vi "Unsubscribe.vi"(8 "error in (no error)":errorcluster, 11 "Subscription":refnum<class "Subscription.lvclass">) -> (0 "error out":errorcluster)   [LabVIEW 2015, in "NI_AWS_SNS.lvlib" / "Subscription.lvclass"]
doc: "Deletes a subscription.\n\nThis action is throttled at 100 transactions per second (TPS)."
uses:
  Subscription.lvclass
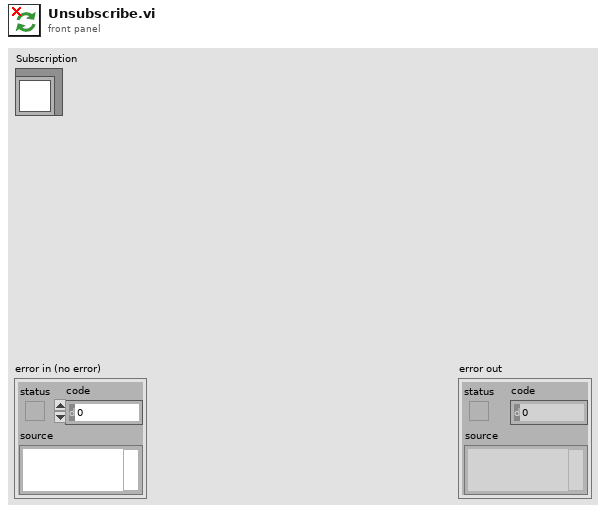
[diagram p1: front panel]
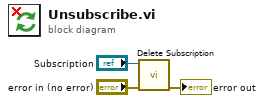
[diagram p0: block diagram]
diagram:
  n1 = call "Delete Subscription.vi"("error in (no error)"="error in (no error)", "Subscription"="Subscription") -> ("error out"=→"error out":errorcluster)  [unwired: 9 in]
